vi "single frame module.vi"(7 "Channel":u32(ring)=1 items=["A"=1, "B"=2, "A + B"=3, "C"=4, "A + C"=5, "A + B"=6, "D"=8, "A + D"=9, "B + D"=10, "C + D"=12, "A + B + C + D"=15], 8 "Error in":errorcluster, 10 "Scan Type in":T1, 11 "Scan Status in":enum16{"Start", "Continue Scan", "Finish Scan"}(ring)) -> (0 "Error Out":errorcluster)   [LabVIEW 2018]
uses:
  Controls/ScanType.ctl
  Controls/QueueNames.ctl
  Controls/MessagePacket.ctl
  Controls/Queue Manager Actions.ctl
  Controls/FGV Actions.ctl
panel:
  in  "max queue size (-1, unlimited)":i32=10
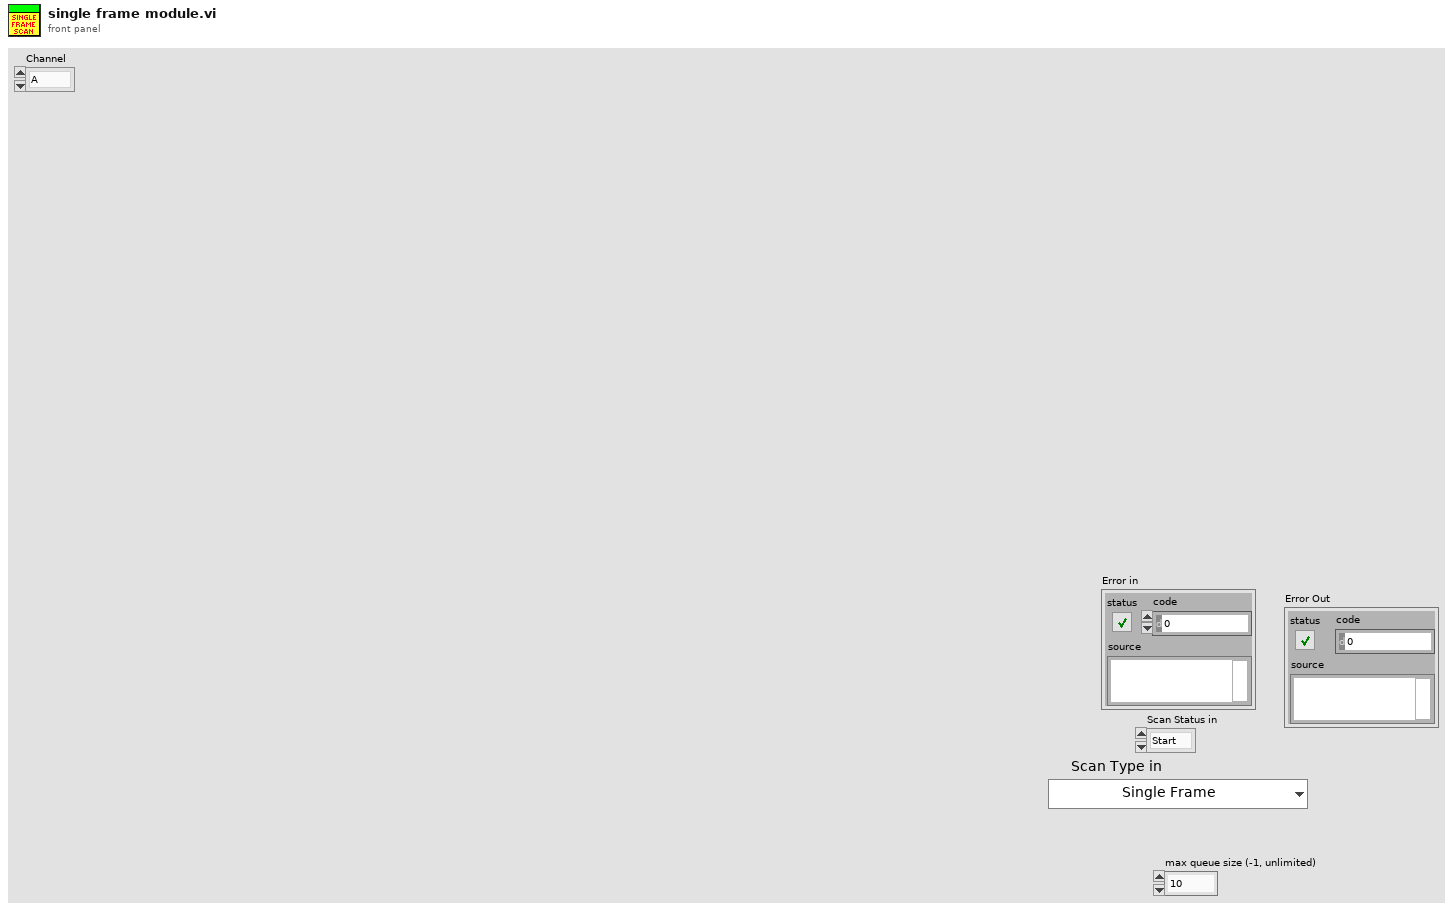
[diagram p1: front panel]
types:
  T1 = typedef "ScanType.ctl" = enum16{"Single Frame", "Continuous Frame", "ROI Line", "Vibratome", "Mosaic", "Mosaic + Slice"}
  T2 = typedef "Queue Manager Actions.ctl" = enum16{"Init", "Enqueue", "Enqueue All", "Preview Queue", "Dequeue", "Get Status", "Flush Queue", "Flush All Queues", "Release All Queues", "Release Queue", "Enqueue at Opposite End"}
  T3 = typedef "MessagePacket.ctl" = cluster{"Message":string, "Parameter":variant}
  T4 = typedef "QueueNames.ctl" = enum16{"Main GUI", "Main Scan Processor", "Main Processing", "Main Saving", "Main Display", "Main Table Stage GUI", "Main Table Stage Proc.", "Scan Engine", "Vibratome GUI", "Vibratome Processor", "Slice Engine"}
  T5 = typedef "FGV Actions.ctl" = enum16{"Init", "Set", "Get", "Clear"}
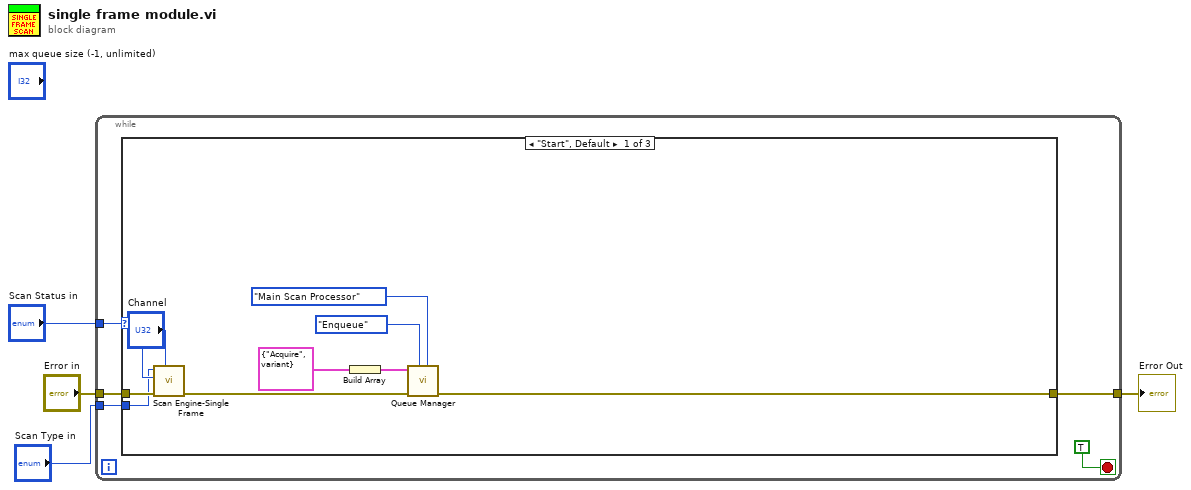
[diagram p0: block diagram]
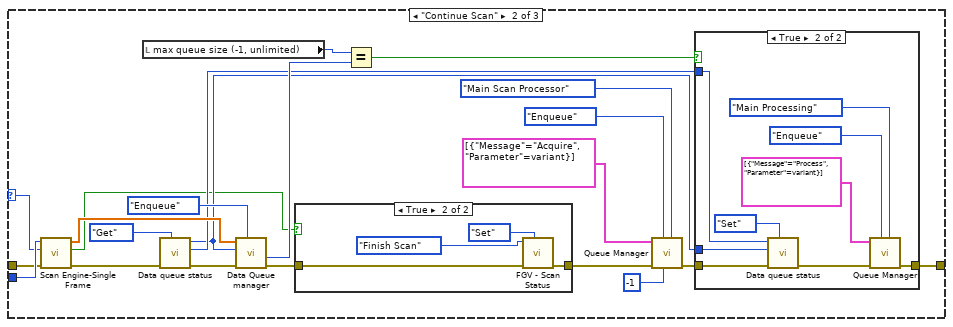
[diagram p2: hidden frame]
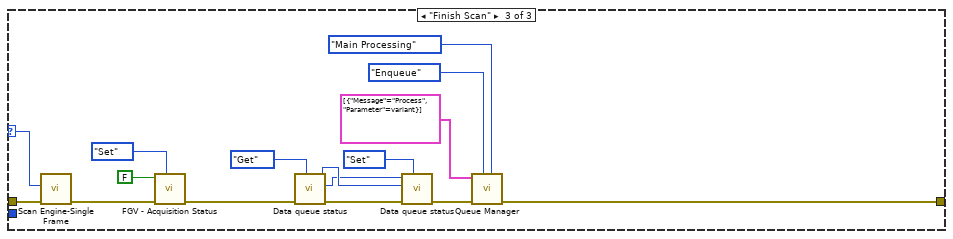
[diagram p5: hidden frame]
diagram:
  n1 = while {
    tunnel: "Error in" -> [w8]
    tunnel: "Scan Status in" -> [w7]
    tunnel: "Scan Type in" -> [w6]
    tunnel: [w5] -> w1
    stop <- TRUE stop-if-true
    n2 = case shown="\"Start\", Default" w7 {
      selector: w7 -> [w18 w33 w72]
      tunnel: w6 -> [w17 w41 _]
      tunnel: w8 -> [w19 w40 w71]
      tunnel: [w12 w25 w64] -> w5
      frame "Start", Default {
        n3 = call "Scan Engine-Single Frame.vi"("Channel"="Channel", "Error in"=w19, "Scan Status"=w18, "Scan Type in"=w17) -> ("Error Out"=w13:errorcluster)  [unwired: 5 in, 2 out]
        n4 = Build Array(T3 {"Message"="Acquire", "Parameter"=variant} ("Message Packet [In]")) -> (w14:T3[])
        n5 = call "Queue Manager.vi"("Queue Name"=QueueNames."Main Scan Processor", "Action"=Queue_Manager_Actions."Enqueue", "Error In"=w13, "Message Packet Array"=w14) -> ("Error Out"=w12:errorcluster)  [unwired: 3 in, 4 out]
      }
      frame "Continue Scan" {
        n6 = call "Scan Engine-Single Frame.vi"("Error in"=w40, "Scan Status"=w33, "Scan Type in"=w41) -> ("Error Out"=w32:errorcluster, "task done?"=w20:bool, "data out"=w34:sgl[])  [unwired: 6 in]
        n7 = local read "max queue size (-1, unlimited)"() -> (w28:i32)
        n8 = call "Data queue status.vi"("action"=enum16{"Init", "Get", "Set"}."Get", "error in"=w32) -> ("error out"=w31:errorcluster, "dequeue channel"=w24:enum16{"1", "2"}, "enqueue channel"=w23:enum16{"1", "2"})  [unwired: 7 in]
        n9 = call "Data Queue manager.vi"("Action"=Queue_Manager_Actions."Enqueue", "error in"=w31, "enqueue channel"=w23, "Buffer"=w34) -> ("error out"=w22:errorcluster, "# elements in queue"=w29:i32)  [unwired: 4 in, 2 out]
        n10 = case shown="True" w20 {
          tunnel: w22 -> [w42 w45]
          tunnel: [w42 w44] -> w21
          frame False {
          }
          frame True {
            n11 = call "FGV - Scan Status.vi"("Actions"=FGV_Actions."Set", "Error In"=w45, "Scan Status in"=enum16{"Start", "Continue Scan", "Finish Scan"}."Finish Scan") -> ("Error Out"=w44:errorcluster)  [unwired: 6 in, 2 out]
          }
        }
        n12 = Equal?(x=w28, y=w29) -> (x = y?=w27:bool)
        n13 = call "Queue Manager.vi"("Queue Name"=QueueNames."Main Scan Processor", "timeout in ms (-1)"=-1, "Action"=Queue_Manager_Actions."Enqueue", "Error In"=w21, "Message Packet Array"=T3[] [{"Message"="Acquire", "Parameter"=variant}] ("Message Packet [In]")) -> ("Error Out"=w26:errorcluster)  [unwired: 2 in, 4 out]
        n14 = case shown="True" w27 {
          tunnel: [w47 w51] -> w25
          tunnel: w26 -> [w47 w49]
          tunnel: w24 -> [_ w55]
          tunnel: w23 -> [_ w54]
          frame False {
          }
          frame True {
            n15 = call "Data queue status.vi"("action"=enum16{"Init", "Get", "Set"}."Set", "error in"=w49, "dequeue channel"=w54, "enqueue channel"=w55) -> ("error out"=w48:errorcluster)  [unwired: 5 in, 2 out]
            n16 = call "Queue Manager.vi"("Queue Name"=QueueNames."Main Processing", "Action"=Queue_Manager_Actions."Enqueue", "Error In"=w48, "Message Packet Array"=T3[] [{"Message"="Process", "Parameter"=variant}]) -> ("Error Out"=w51:errorcluster)  [unwired: 3 in, 4 out]
          }
        }
      }
      frame "Finish Scan" {
        n17 = call "Scan Engine-Single Frame.vi"("Error in"=w71, "Scan Status"=w72) -> ("Error Out"=w68:errorcluster)  [unwired: 7 in, 2 out]
        n18 = call "FGV - Acquisition Status.vi"("Actions"=FGV_Actions."Set", "Error In"=w68, "Status In"=FALSE) -> ("Error Out"=w61:errorcluster)  [unwired: 6 in, 2 out]
        n19 = call "Data queue status.vi"("action"=enum16{"Init", "Get", "Set"}."Get", "error in"=w61) -> ("error out"=w60:errorcluster, "dequeue channel"=w57:enum16{"1", "2"}, "enqueue channel"=w58:enum16{"1", "2"})  [unwired: 7 in]
        n20 = call "Data queue status.vi"("action"=enum16{"Init", "Get", "Set"}."Set", "error in"=w60, "dequeue channel"=w58, "enqueue channel"=w57) -> ("error out"=w59:errorcluster)  [unwired: 5 in, 2 out]
        n21 = call "Queue Manager.vi"("Queue Name"=QueueNames."Main Processing", "Action"=Queue_Manager_Actions."Enqueue", "Error In"=w59, "Message Packet Array"=T3[] [{"Message"="Process", "Parameter"=variant}]) -> ("Error Out"=w64:errorcluster)  [unwired: 3 in, 4 out]
      }
    }
  }
  "Error Out" <- w1
